vi "Set XY Accleration.vi"(8 "error in (no error)":errorcluster, 10 "mm/s":dbl format="%#_13g", 11 "Motion in":refnum<class "Motion.lvclass">) -> (0 "error out":errorcluster, 3 "Motion out":refnum<class "Motion.lvclass">)   [LabVIEW 2018, in "Motion.lvclass"]
uses:
  Motion.lvclass
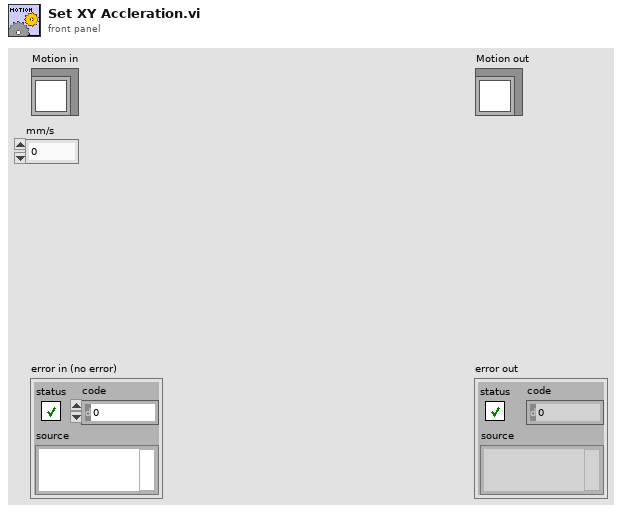
[diagram p1: front panel]
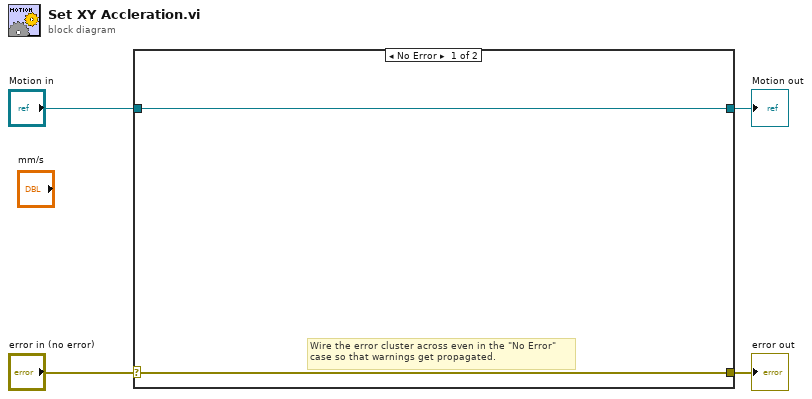
[diagram p0: block diagram]
diagram:
  n1 = case shown="No Error" "error in (no error)" {
    selector: "error in (no error)" -> [w5 w8]
    tunnel: [w5 w8] -> w3
    tunnel: [w6 w7] -> w1
    tunnel: "Motion in" -> [w6 w7]
    frame No Error {
      # "Wire the error cluster across even in the \"No Error\"\ncase so that warnings get propagated."
    }
    frame Error {
    }
  }
  "error out" <- w3
  "Motion out" <- w1
